vi "Read States.vi"(8 "error in (no error)":errorcluster, 11 "CSM-Helper in":refnum<class "CSM-Helper.lvclass">) -> (0 "error out":errorcluster, 2 "Value":string[](array[string]), 3 "CSM-Helper out":refnum<class "CSM-Helper.lvclass">)   [LabVIEW 2017, in "CSM-Helper.lvclass"]
doc: "### Read States.vi\n\n-- <b>Controls</b> --\n- <b>CSM-Helper in</b>: CSMHelper input\n\n-- <b>Indicators</b> --\n- <b>Value</b>:\n- <b>CSM-Helper out</b>: CSMHelper output"
uses:
  CSM-Helper.lvclass
  CSM-Helper.lvclass/CSM-Helper.ctl
  _Shared/CSM Shared.lvlib
  Communicable State Machine.lvlib
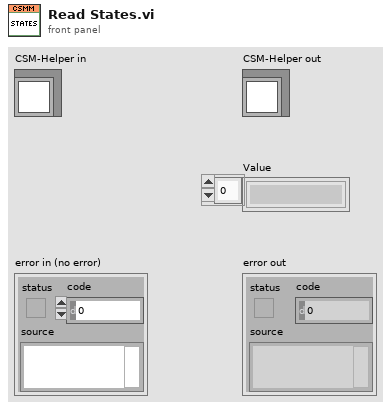
[diagram p1: front panel]
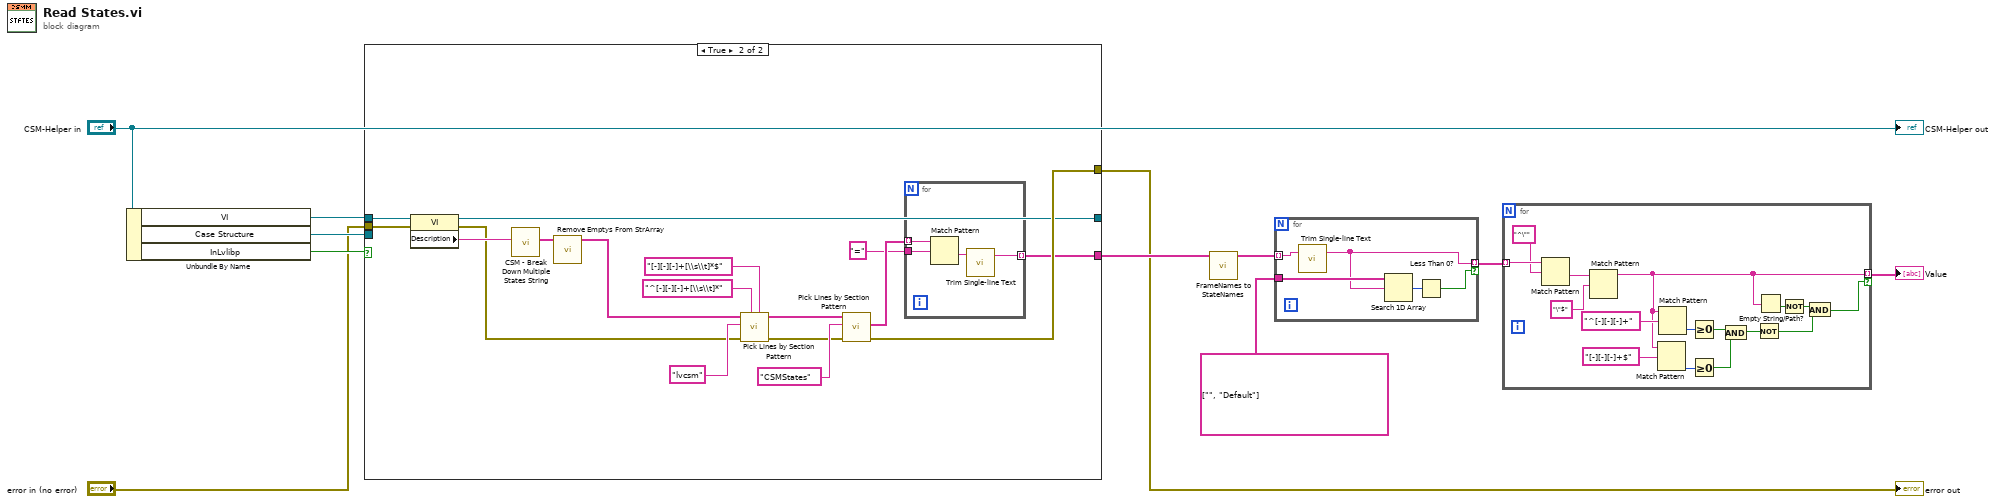
[diagram p0: block diagram]
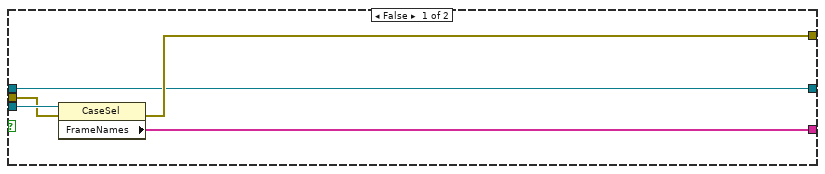
[diagram p2: hidden frame]
diagram:
  n1 = Unbundle By Name("CSM-Helper in") -> ("VI"=w4:refnum<vi>, "Case Structure"=w6:refnum<vi>, "InLvlibp"=w5:bool)
  n2 = case shown="True" w5 {
    tunnel: w6 -> [w16 _]
    tunnel: [w13 w27] -> w2
    tunnel: [w14 w30] -> w1
    tunnel: "error in (no error)" -> [w15 w31]
    tunnel: w4 -> [w12 w32]
    tunnel: [w12 w17] -> _
    frame False {
      n3 = property on="Property Node" class="CaseSel"(reference=w16, error in=w15) -> (error out=w14:errorcluster, "FrameNames"=w13:string[])  [unwired: 1 out]
    }
    frame True {
      n4 = property class="VI"(reference=w32, error in=w31) -> (reference out=w17:refnum<vi>, error out=w24:errorcluster, "Description"=w25:string)
      n5 = call "CSM - Break Down Multiple States String.vi"("States"=w25) -> ("Multiple States"=w19:string[])  [unwired: 10 in]
      n6 = call "Remove Emptys From StrArray.vi"("Array In"=w19) -> ("Array Out"=w18:string[])  [unwired: 10 in]
      n7 = call "Pick Lines by Section Pattern.vi"("RegExp Right(\"^[\")"="[-][-][-]+[\\s\\t]*$" ("RegExp Lef(\"^[\")"), "RegExp Lef(\"^[\")"="^[-][-][-]+[\\s\\t]*" ("RegExp Lef(\"^[\")"), "error in (no error)"=w24, "Session Name"="lvcsm" ("[] Session Name"), "Config Text List"=w18) -> ("error out"=w23:errorcluster, "Config Text List out"=w22:string[])  [unwired: 2 in, 3 out]
      n8 = call "Pick Lines by Section Pattern.vi"("error in (no error)"=w23, "Session Name"="CSMStates" ("[] Session Name"), "Config Text List"=w22) -> ("error out"=w30:errorcluster, "Session"=w29:string[])  [unwired: 4 in, 3 out]
      n9 = for {
        tunnel: w29 -> [w37] mode=indexing
        tunnel: "=" ("regular expression") -> [w36]
        tunnel: [w34] -> w27 mode=indexing
        n10 = Match Pattern(string=w37, regular expression=w36) -> (after substring=w35:string)  [unwired: 1 in, 3 out]
        n11 = call "Trim Single-line Text.vi"("single-line text"=w35) -> ("trimed text"=w34:string)  [unwired: 2 in]
      }
    }
  }
  "error out" <- w1
  n12 = call "FrameNames to StateNames.vi"("FrameNames"=w2) -> ("Array of Strings"=w7:string[])  [unwired: 10 in]
  n13 = for {
    tunnel: w7 -> [w42] mode=indexing
    tunnel: [w40] -> w11 mode=indexing if=w38
    tunnel: string[] ["", "Default"] ("items to filter") -> [w41]
    n14 = call "Trim Single-line Text.vi"("single-line text"=w42) -> ("trimed text"=w40:string)  [unwired: 2 in]
    n15 = Search 1D Array(1D array=w41, element=w40) -> (index of element=w39:i32)  [unwired: 1 in]
    n16 = Less Than 0?(x=w39) -> (x < 0?=w38:bool)
  }
  n17 = for {
    tunnel: w11 -> [w58] mode=indexing
    tunnel: [w43] -> w9 mode=indexing if=w47
    n18 = Match Pattern(string=w58, regular expression="^\"") -> (after substring=w56:string)  [unwired: 1 in, 3 out]
    n19 = Match Pattern(string=w56, regular expression="\"$") -> (before substring=w43:string)  [unwired: 1 in, 3 out]
    n20 = Match Pattern(string=w43, regular expression="[-][-][-]+$") -> (offset past match=w51:i32)  [unwired: 1 in, 3 out]
    n21 = Match Pattern(string=w43, regular expression="^[-][-][-]+") -> (offset past match=w52:i32)  [unwired: 1 in, 3 out]
    n22 = Greater Or Equal To 0?(x=w52) -> (x >= 0?=w50:bool)
    n23 = Greater Or Equal To 0?(x=w51) -> (x >= 0?=w49:bool)
    n24 = And(x=w50, y=w49) -> (x .and. y?=w48:bool)
    n25 = Not(x=w48) -> (.not. x?=w46:bool)
    n26 = Empty String/Path?(string/path=w43) -> (empty?=w45:bool)
    n27 = Not(x=w45) -> (.not. x?=w44:bool)
    n28 = And(x=w44, y=w46) -> (x .and. y?=w47:bool)
  }
  "Value" <- w9
  "CSM-Helper out" <- "CSM-Helper in"
